vi "P4CMDSub Get Config Info.vi"(6 "operation message":string, 8 "error in (no error)":errorcluster, 11 "source control reference in":T1) -> (0 "error out":errorcluster, 1 "port":string, 2 "user":string, 3 "source control reference out":T1, 5 "client":string)   [LabVIEW 2017, in "NI_SCC_P4CMD.lvlib"]
uses:
  <vilib>/SourceControl/Providers/P4CMD/NI_SCC_P4CMD.lvlib
  <vilib>/SourceControl/sccapi/SCCAPI Refnum.ctl
  <vilib>/SourceControl/Providers/P4CMD/P4CMD Mgr Functions.ctl
  <vilib>/SourceControl/sccapi/NI_SCC.lvlib
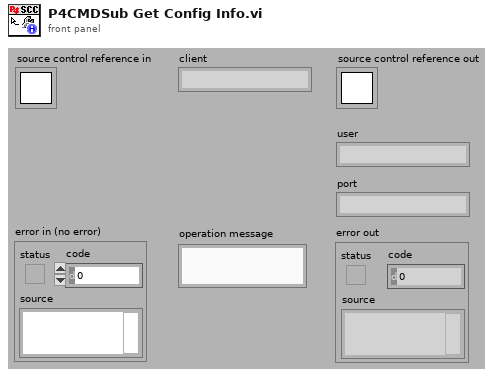
[diagram p1: front panel]
types:
  T1 = typedef "NI_SCC.lvlib/SCCAPI Refnum.ctl" = refnum<k1>
  T2 = typedef "NI_SCC_P4CMD.lvlib/P4CMD Mgr Functions.ctl" = enum16{"Init", "Open", "Set Config Opts", "Initialized?", "IsRefValid?", "Get Config Opts", "Get Global Commands", "Close", "Uninit"}
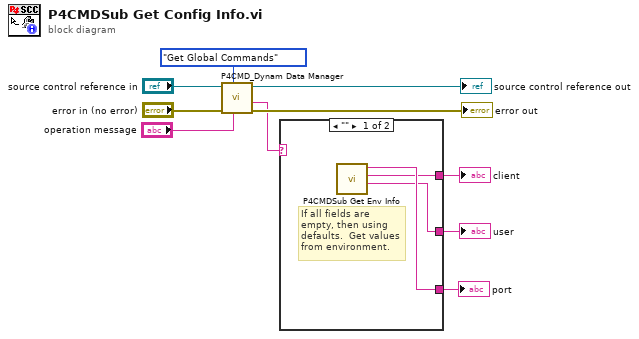
[diagram p0: block diagram]
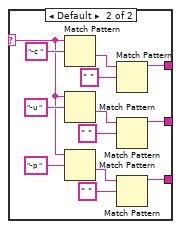
[diagram p2: hidden frame]
diagram:
  n1 = call <vilib>:"P4CMD_Dynam Data Manager.vi"("operation message"="operation message", "function"=P4CMD_Mgr_Functions."Get Global Commands", "error in (no error)"="error in (no error)", "source control reference in"="source control reference in") -> ("error out"=→"error out":errorcluster, "global commands"=w1:string, "source control reference out"=→"source control reference out":T1)  [unwired: 2 in, 3 out]
  n2 = case shown="\"\"" w1 {
    selector: w1 -> [_ w14]
    tunnel: [w12 w20] -> w8
    tunnel: [w11 w19] -> w7
    tunnel: [w13 w18] -> w6
    frame "" {
      # "If all fields are empty, then using defaults.  Get values from environment."
      n3 = call <vilib>:"P4CMDSub Get Env Info.vi"() -> ("user"=w11:string, "client"=w12:string, "port"=w13:string)  [unwired: 8 in, 1 out]
    }
    frame Default {
      n4 = Match Pattern(string=w14, regular expression="-c ") -> (after substring=w24:string)  [unwired: 1 in, 3 out]
      n5 = Match Pattern(string=w14, regular expression="-u ") -> (after substring=w21:string)  [unwired: 1 in, 3 out]
      n6 = Match Pattern(string=w14, regular expression="-p ") -> (after substring=w17:string)  [unwired: 1 in, 3 out]
      n7 = Match Pattern(string=w24, regular expression=" ") -> (before substring=w20:string)  [unwired: 1 in, 3 out]
      n8 = Match Pattern(string=w21, regular expression=" ") -> (before substring=w19:string)  [unwired: 1 in, 3 out]
      n9 = Match Pattern(string=w17, regular expression=" ") -> (before substring=w18:string)  [unwired: 1 in, 3 out]
    }
  }
  "client" <- w8
  "user" <- w7
  "port" <- w6
